vi "dlgMagPhasePlot.vi"(8 "error in (no error)":errorcluster, 11 "AllData":T1 {"FlukeData"."DataAnalysisArray"."TimeStamp" format="%^<%.3X\n%x>T"; "FlukeData"."ModelDataArray"."FREQUENCY" format="%#_6f"; "FlukeData"."ModelDataArray"."TimeStamp" format="%^<%.3X\n%x>T"; "FlukeData"."PMUDataArray"."FREQUENCY" format="%#_6f"; "FlukeData"."PMUDataArray"."TimeStamp" format="%^<%.3X\n%x>T"; "NISTData"."DataAnlysisArray"."Time" format="%.6f"; "NISTData"."DataAnlysisArray"."TimeStamp" format="%^<%.3X\n%x>T"; "NISTData"."DUTDataArray"."TimeStamp" format="%^<%.3X\n%x>T"; "NISTData"."DUTDataArray"."Time" format="%.6f"; "NISTData"."NIDataArray"."TimeStamp" format="%^<%.3X\n%x>T"; "NISTData"."NIDataArray"."Time" format="%.6f"}) -> (0 "error out":errorcluster)   [LabVIEW 2014]
uses:
  typedefs/PlotSource.ctl
  typedefs/Alldata.ctl
  typedefs/NISTData.ctl
  typedefs/NIDataArray.ctl
  typedefs/NIData.ctl
  typedefs/PhasorRectangular.ctl
  typedefs/DUTData.ctl
  typedefs/NICalcAnalysis.ctl
  typedefs/CalcPhasorError.ctl
  typedefs/PlotDataArrays.ctl
  typedefs/PmuRawDataCluster.ctl
  typedefs/CalcAnalysis.ctl
  typedefs/eMainAction.ctl
panel:
  in  "btnExit":bool
  in  "PlotSource":T12
  out "Phase Plot":T13(graph)
  out "Mag Plot":T13(graph)
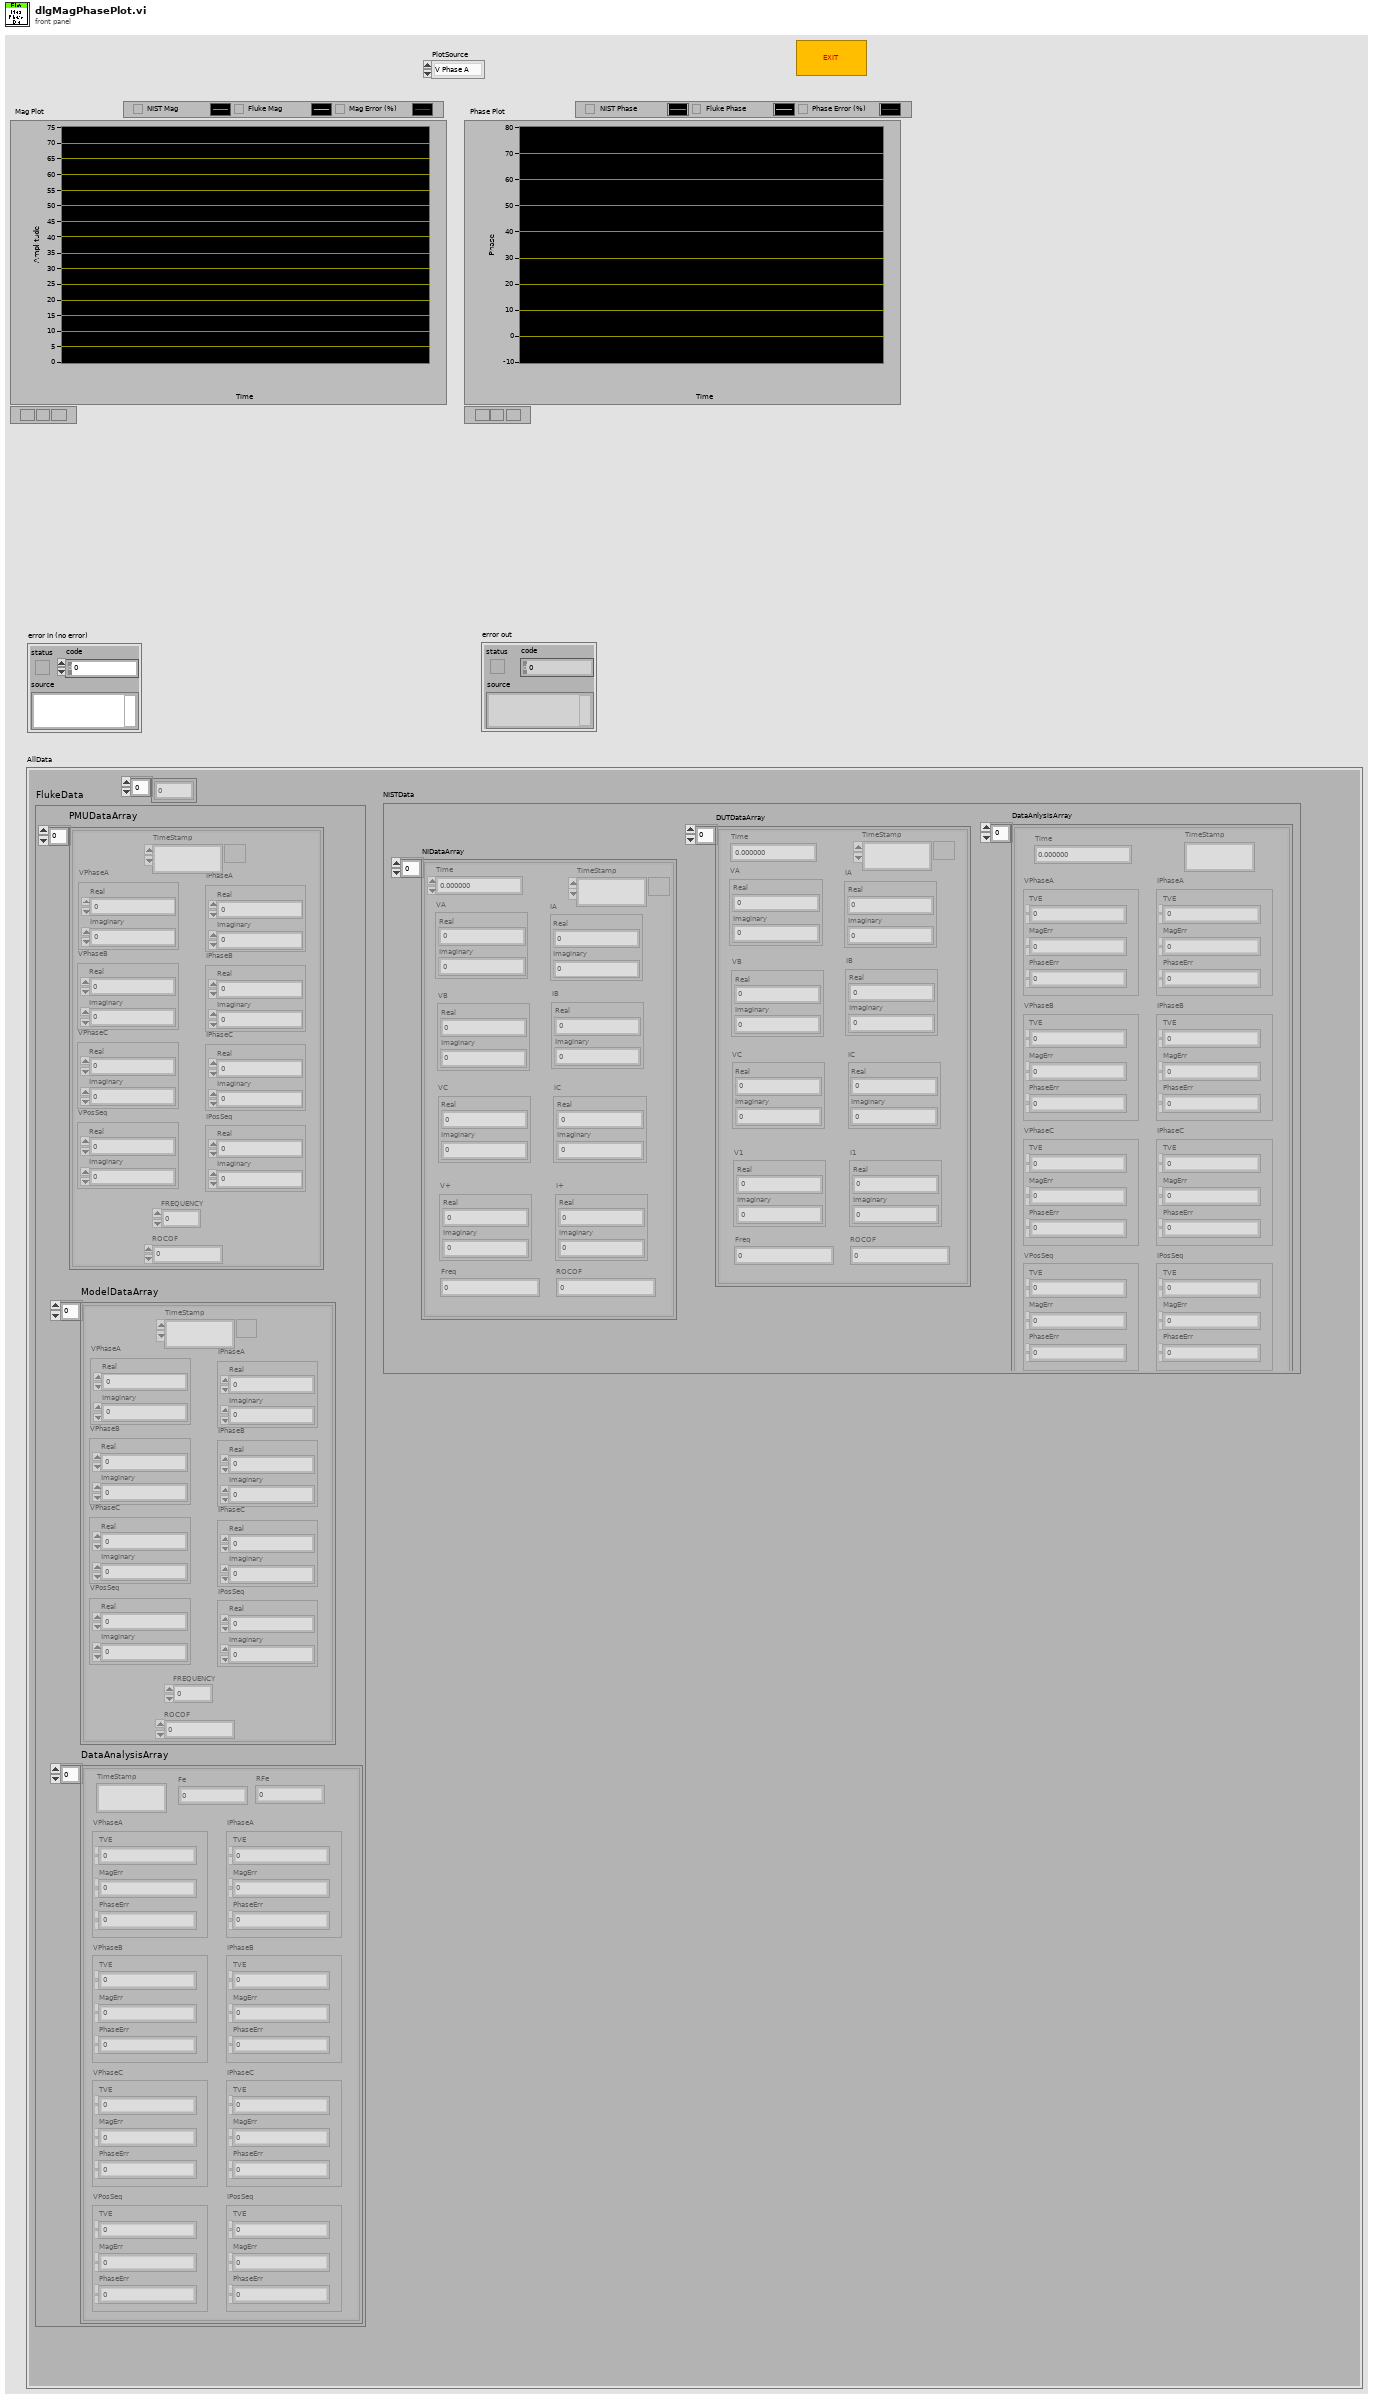
[diagram p1: front panel]
types:
  T1 = typedef "Alldata.ctl" = cluster{"NISTData":T2, "FlukeData":T9, "Params":dbl[]}
  T2 = typedef "NISTData.ctl" = cluster{"NIDataArray":T3, "DUTDataArray":T6[], "DataAnlysisArray":T7[]}
  T3 = typedef "NIDataArray.ctl" = T4[]
  T4 = typedef "NIData.ctl" = cluster{"Time":dbl, "VA":T5, "VB":T5, "VC":T5, "V+":T5, "IA":T5, "IB":T5, "IC":T5, "I+":T5, "Freq":dbl, "ROCOF":dbl, "TimeStamp":timestamp}
  T5 = typedef "PhasorRectangular.ctl" = cluster{"Real":dbl, "Imaginary":dbl}
  T6 = typedef "DUTData.ctl" = cluster{"Time":dbl, "VA":T5, "VB":T5, "VC":T5, "V1":T5, "IA":T5, "IB":T5, "IC":T5, "I1":T5, "Freq":dbl, "ROCOF":dbl, "TimeStamp":timestamp}
  T7 = typedef "NICalcAnalysis.ctl" = cluster{"Time":dbl, "VPhaseA":T8, "VPhaseB":T8, "VPhaseC":T8, "VPosSeq":T8, "IPhaseA":T8, "IPhaseB":T8, "IPhaseC":T8, "IPosSeq":T8, "Fe":dbl, "RFe":dbl, "TimeStamp":timestamp}
  T8 = typedef "CalcPhasorError.ctl" = cluster{"TVE":dbl, "MagErr":dbl, "PhaseErr":dbl}
  T9 = typedef "PlotDataArrays.ctl" = cluster{"PMUDataArray":T10[], "ModelDataArray":T10[], "DataAnalysisArray":T11[]}
  T10 = typedef "PmuRawDataCluster.ctl" = cluster{"TimeStamp":timestamp, "VPhaseA":T5, "VPhaseB":T5, "VPhaseC":T5, "VPosSeq":T5, "IPhaseA":T5, "IPhaseB":T5, "IPhaseC":T5, "IPosSeq":T5, "FREQUENCY":dbl, "ROCOF":sgl}
  T11 = typedef "CalcAnalysis.ctl" = cluster{"TimeStamp":timestamp, "VPhaseA":T8, "VPhaseB":T8, "VPhaseC":T8, "VPosSeq":T8, "IPhaseA":T8, "IPhaseB":T8, "IPhaseC":T8, "IPosSeq":T8, "Fe":dbl, "RFe":dbl}
  T12 = typedef "PlotSource.ctl" = enum16{"V Phase A", "V Phase B", "V Phase C", "I Phase A", "I Phase B", "I Phase C"}
  T13 = cluster{"TimestampArray":timestamp[], "Y":dbl[]}[]
  T14 = typedef "eMainAction.ctl" = enum16{"Init", "ProcessUI", "Exit"}
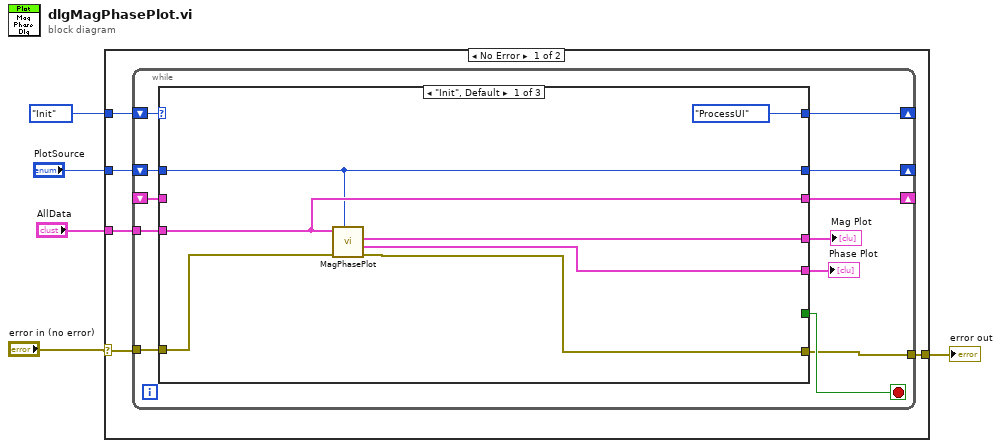
[diagram p0: block diagram]
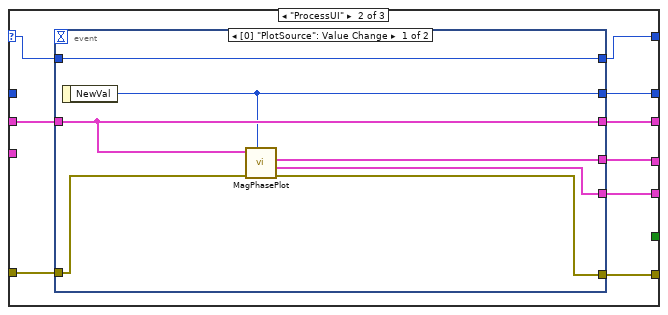
[diagram p2: hidden frame]
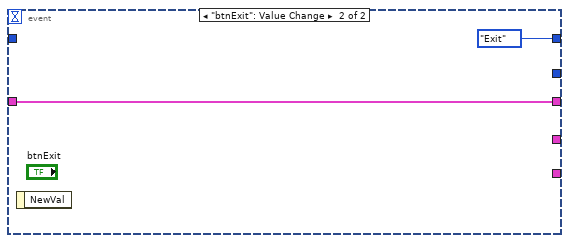
[diagram p3: hidden frame]
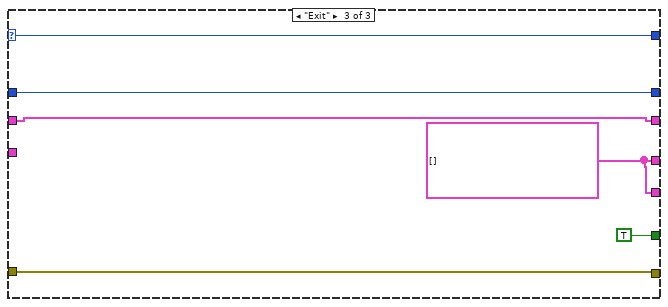
[diagram p4: hidden frame]
diagram:
  n1 = case shown="No Error" "error in (no error)" {
    selector: "error in (no error)" -> [w6 w54]
    tunnel: "AllData" -> [w10 _]
    tunnel: eMainAction."Init" ("eMainAction") -> [w9 _]
    tunnel: "PlotSource" -> [w8 _]
    tunnel: [w7 w54] -> w2
    frame No Error {
      n2 = while {
        tunnel: w10 -> [w22]
        shift-right: [w20] -> _
        shift-left: w9 -> [w21]
        shift-right: [w19] -> _
        shift-left: _ -> [w14]
        shift-right: [w17] -> _
        shift-left: w8 -> [w18]
        tunnel: w6 -> [w12]
        tunnel: [w11] -> w7
        stop <- w13 stop-if-true
        n3 = case shown="\"Init\", Default" w21 {
          selector: w21 -> [_ w38 w50]
          tunnel: w22 -> [w28 _ _]
          tunnel: [eMainAction."ProcessUI" ("eMainAction") w37 w50] -> w20
          tunnel: [w28 w33 w49] -> w19
          tunnel: w18 -> [w27 _ w51]
          tunnel: [w27 w32 w51] -> w17
          tunnel: [w26 w35 w52] -> w16
          tunnel: [w25 w34 w52] -> w15
          tunnel: w14 -> [_ w36 w49]
          tunnel: [_ _ TRUE] -> w13
          tunnel: w12 -> [w24 w31 w48]
          tunnel: [w23 w30 w48] -> w11
          frame "Init", Default {
            n4 = call "MagPhasePlot.vi"("PlotSource"=w27, "error in (no error)"=w24, "AllData"=w28) -> ("error out"=w23:errorcluster, "Phase Plot"=w25:T13, "Mag Plot"=w26:T13)  [unwired: 6 in]
          }
          frame "ProcessUI" {
            n5 = event shown="[0] \"PlotSource\": Value Change" {
              selector: _ -> [_ _]
              dyn-events: _ -> [_ _]
              timeout: _ -> [_ _]
              tunnel: w38 -> [w45 _]
              tunnel: [w45 eMainAction."Exit" ("eMainAction")] -> w37
              tunnel: w36 -> [w42 w46]
              tunnel: [w44 _] -> w35
              tunnel: [w43 _] -> w34
              tunnel: [w42 w46] -> w33
              tunnel: [w41 _] -> w32
              tunnel: w31 -> [w40 _]
              tunnel: [w39 _] -> w30
              event Value Change {
                n6 = event-data() -> ("NewVal"=w41:T12)  [unwired: 1 in]
                n7 = call "MagPhasePlot.vi"("PlotSource"=w41, "error in (no error)"=w40, "AllData"=w42) -> ("error out"=w39:errorcluster, "Phase Plot"=w43:T13, "Mag Plot"=w44:T13)  [unwired: 6 in]
              }
              event "btnExit": Value Change {
                n8 = event-data() -> ()  [unwired: 1 in, 1 out]
              }
            }
          }
          frame "Exit" {
            w52 = T13 [] ("Mag Plot")
          }
        }
        "Phase Plot" <- w15
        "Mag Plot" <- w16
      }
    }
    frame Error {
    }
  }
  "error out" <- w2
